vi "create_folder.vi"(8 "error in":errorcluster, 9 "FolderName":string, 11 "main path":path) -> (0 "error out":errorcluster, 1 "Created":bool, 3 "path out":path)   [LabVIEW 2018]
panel:
  out "folder names":string[](array[string])
  out "filenames":string[](array[string])
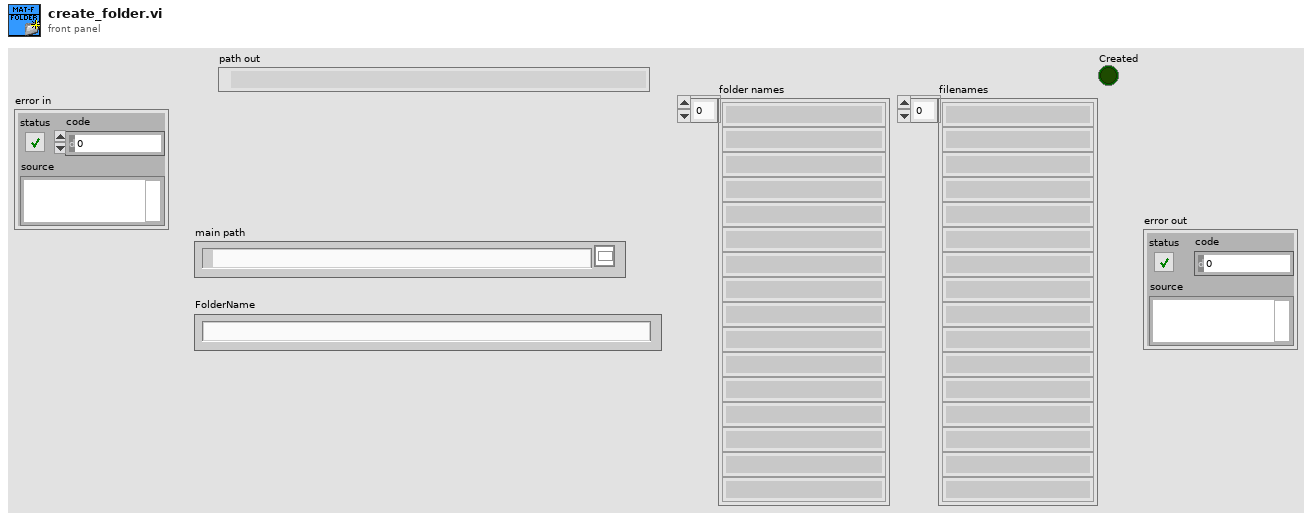
[diagram p1: front panel]
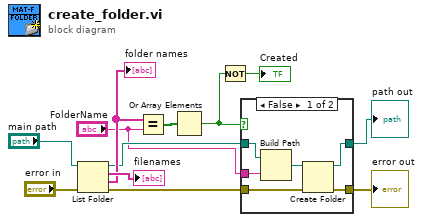
[diagram p0: block diagram]
diagram:
  n1 = List Folder(path="main path", error in="error in") -> (path out=w6:path, filenames=→"filenames":string[], folder names=w9:string[], error out=w5:errorcluster)  [unwired: 2 in]
  "folder names" <- w9
  n2 = Equal?(x=w9, y="FolderName") -> (x = y?=w8:bool[])
  n3 = Or Array Elements(Boolean array=w8) -> (logical OR=w1:bool)
  n4 = Not(x=w1) -> (.not. x?=→"Created":bool)
  n5 = case shown="False" w1 {
    tunnel: [w14 w20] -> w7
    tunnel: w6 -> [w18 w20]
    tunnel: w5 -> [w16 w19]
    tunnel: [w13 w19] -> w3
    tunnel: "FolderName" -> [w15 _]
    frame False {
      n6 = Build Path(base path=w18, name or relative path=w15) -> (appended path=w17:path)
      n7 = Create Folder(path (use dialog)=w17, error in=w16) -> (created path=w14:path, error out=w13:errorcluster)  [unwired: 1 in, 1 out]
    }
    frame True {
    }
  }
  "path out" <- w7
  "error out" <- w3
